vi "GetHiSpeedDeviceNameLocIDChannel.vi"(5 "error in (no error)":errorcluster, 6 "Device index":u32) -> (0 "error out":errorcluster, 1 "Location ID":u32, 2 "Result":u32, 3 "Channel":string, 4 "Device name":string)   [LabVIEW 2010]
uses:
  FTCSPI.dll
panel:
  out "Device type":u32
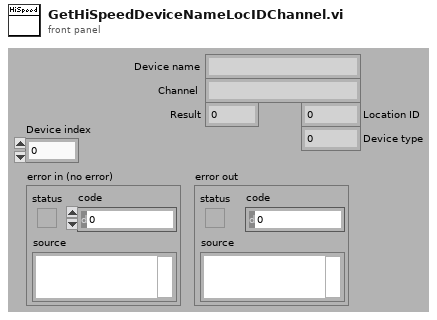
[diagram p1: front panel]
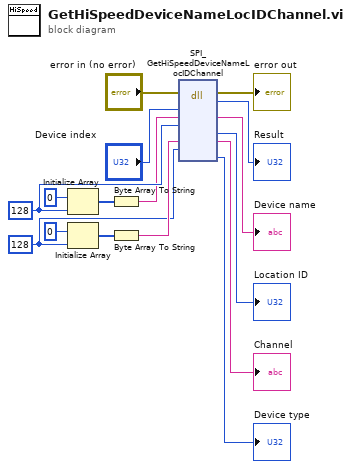
[diagram p0: block diagram]
diagram:
  w2 = 128 ("dimension size")
  w8 = 128 ("dimension size")
  n1 = Initialize Array(u8 0 ("element"), w8) -> (w7:u8[])
  n2 = Initialize Array(u8 0 ("element"), w2) -> (w4:u8[])
  n3 = Byte Array To String(unsigned byte array=w7) -> (string=w6:string)
  n4 = Byte Array To String(unsigned byte array=w4) -> (string=w3:string)
  n5 = dll-call lib="C:/Users/Administrator/Documents/GitHub/labview/FPGA/FTCSPI.dll" fn="SPI_GetHiSpeedDeviceNameLocIDChannel"(error in="error in (no error)", "dwDeviceNameIndex"="Device index", "lpDeviceNameBuffer"=w6, "dwBufferSize"=w8, "lpChannel"=w3, "dwChannelBufferSize"=w2) -> (error out=→"error out":errorcluster, "FTC_STATUS"=→"Result":u32, "lpDeviceNameBuffer"=→"Device name":string, "lpdwLocationId"=→"Location ID":u32, "lpChannel"=→"Channel":string, "lpdwHiSpeedDeviceType"=→"Device type":u32)  [unwired: 7 in, 1 out]
